vi "Test - Add  Property (Enum).vi"() -> ()   [LabVIEW 2020, in "JSON Schema Generator.lvlib"]
uses:
  JSON Schema Generator.lvlib
  <vilib>/addons/_JKI Toolkits/Caraya/classes/Test/Test.lvclass
  <vilib>/addons/_JKI Toolkits/Caraya/classes/Assert/Assert.lvclass
  <vilib>/JDP Science/JSONtext/JSONtext.lvlib
  <vilib>/addons/_JKI Toolkits/Caraya/classes/Assert/Assert Equal Value_Variant.vi
  <vilib>/addons/_JKI Toolkits/Caraya/classes/Assert/Assert Not Error.vi
  Support/Test Enum 2--enum.ctl
panel:
  in  "Test Enum 2":T1
  in  "Test Enum 1":enum16{"Select 1", "Select 2"}(ring)
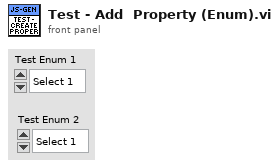
[diagram p1: front panel]
types:
  T1 = typedef "Test Enum 2--enum.ctl" = enum16{"Select 1", "Select 2"}
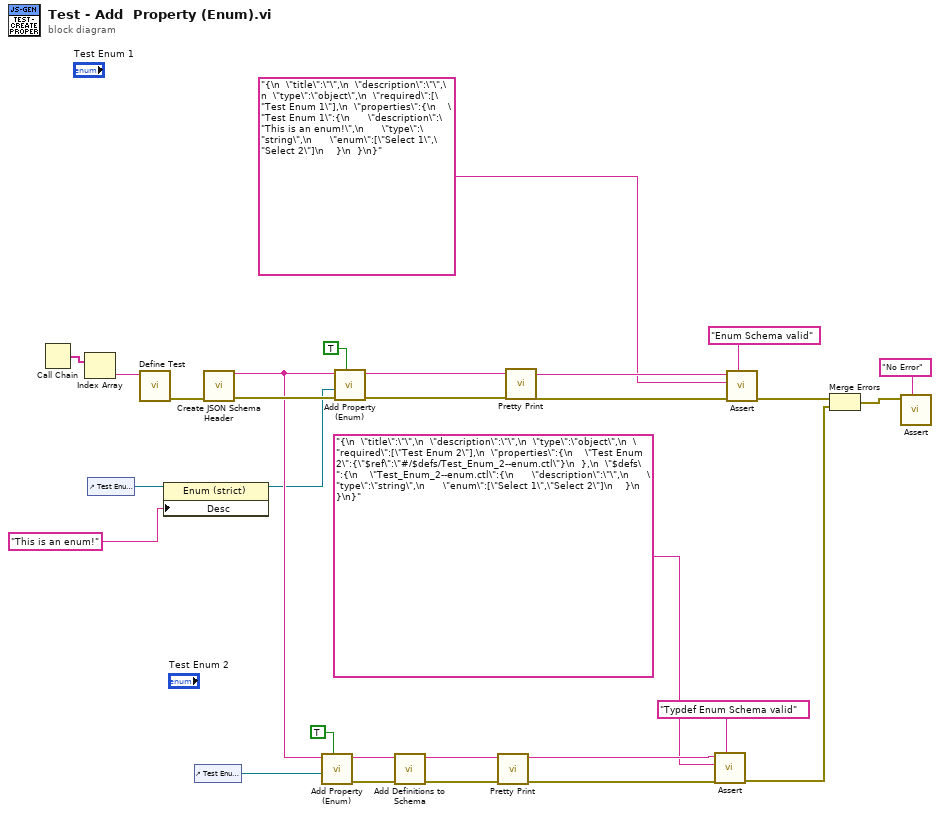
[diagram p0: block diagram]
diagram:
  n1 = Call Chain() -> (call chain=w29:string[])
  n2 = Index Array(array=w29) -> (element=w28:string)  [unwired: 1 in]
  n3 = control-ref of="Test Enum 1"() -> (w17:refnum<vi>)
  n4 = call <vilib>:"Define Test.vi"("Label (VI Title)"=w28) -> ("error out"=w23:errorcluster)  [unwired: 9 in, 1 out]
  n5 = property class="Enum (strict)"(reference=w17, "Desc"="This is an enum!" ("Description")) -> (reference out=w2:refnum<vi>)  [unwired: 1 in, 1 out]
  n6 = control-ref of="Test Enum 2"() -> (w12:refnum<vi>)
  n7 = call "Create JSON Schema Header.vi"("error in (no error)"=w23) -> ("error out"=w16:errorcluster, "JSON Schema out"=w13:string)  [unwired: 9 in]
  n8 = call "Add Property (Enum).vi"("Required?"=TRUE, "Enum In"=w12, "JSON Schema in"=w13) -> ("error out"=w4:errorcluster, "JSON SChema out"=w6:string)  [unwired: 7 in]
  n9 = call "Add Property (Enum).vi"("Required?"=TRUE, "error in (no error)"=w16, "Enum In"=w2, "JSON Schema in"=w13) -> ("error out"=w15:errorcluster, "JSON SChema out"=w18:string)  [unwired: 6 in]
  n10 = call "Add Definitions to Schema.vi"("error in (no error)"=w4, "JSON In"=w6) -> ("error out"=w3:errorcluster, "JSON Out"=w5:string)  [unwired: 8 in]
  n11 = call <vilib>:"Pretty Print.vi"("error in (no error)"=w3, "JSON"=w5) -> ("error out"=w7:errorcluster, "<JSON>"=w10:string)  [unwired: 7 in, 1 out]
  n12 = call <vilib>:"Pretty Print.vi"("error in (no error)"=w15, "JSON"=w18) -> ("error out"=w22:errorcluster, "<JSON>"=w21:string)  [unwired: 7 in, 1 out]
  n13 = call-poly <vilib>:"Assert.vi"("Label"="Typdef Enum Schema valid", "error in (no error)"=w7, "Actual"="{\n  \"title\":\"\",\n  \"description\":\"\",\n  \"type\":\"object\",\n  \"required\":[\"Test Enum 2\"],\n  \"properties\":{\n    \"Test Enum 2\":{\"$ref\":\"#/$defs/Test_Enum_2--enum.ctl\"}\n  },\n  \"$defs\":{\n    \"Test_Enum_2--enum.ctl\":{\n      \"description\":\"\",\n      \"type\":\"string\",\n      \"enum\":[\"Select 1\",\"Select 2\"]\n    }\n  }\n}", "Expected"=w10) -> ("error out"=w8:errorcluster)  [unwired: 6 in, 1 out]
  n14 = call-poly <vilib>:"Assert.vi"("Label"="Enum Schema valid", "error in (no error)"=w22, "Actual"="{\n  \"title\":\"\",\n  \"description\":\"\",\n  \"type\":\"object\",\n  \"required\":[\"Test Enum 1\"],\n  \"properties\":{\n    \"Test Enum 1\":{\n      \"description\":\"This is an enum!\",\n      \"type\":\"string\",\n      \"enum\":[\"Select 1\",\"Select 2\"]\n    }\n  }\n}", "Expected"=w21) -> ("error out"=w26:errorcluster)  [unwired: 6 in, 1 out]
  n15 = Merge Errors(w26, w8) -> (w24:errorcluster)
  n16 = call-poly <vilib>:"Assert.vi"("Label"="No Error", "Not Error?"=w24) -> ()  [unwired: 8 in, 2 out]
